vi "Display_Module.vi"(6 "Start pixel for display":i32=1, 7 "FOV: #A-lines":i32=2048, 8 "error in":errorcluster, 9 "Total pixels to display":i32=500, 10 "Source in":T1) -> (0 "error out":errorcluster, 2 "Image":T1(plugin-control))   [LabVIEW 2018]
uses:
  <vilib>/vision/Image Controls.llb/IMAQ Image.ctl
  Controls/Queue Manager Actions.ctl
  <vilib>/vision/NI_Vision_Development_Module.lvlib
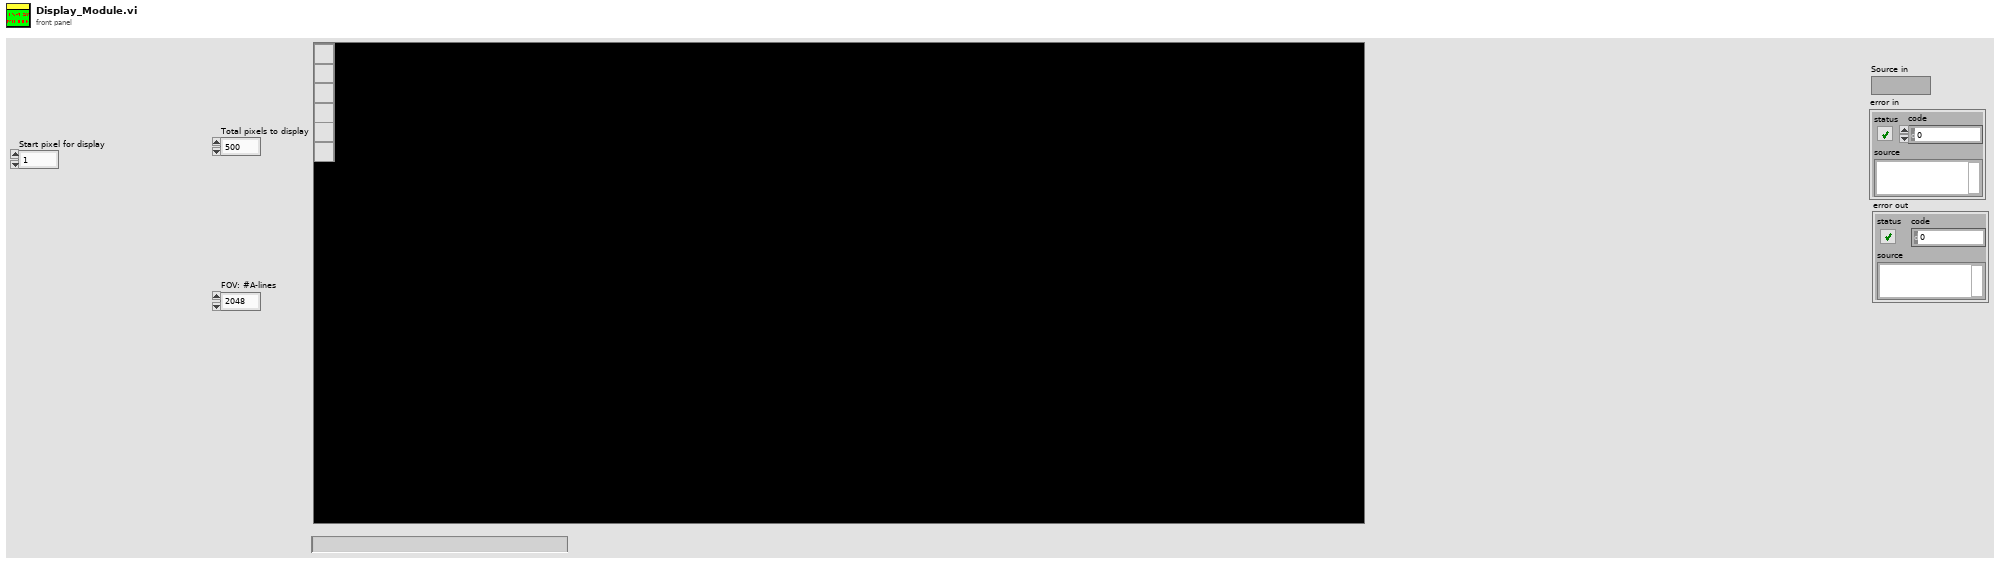
[diagram p1: front panel]
types:
  T1 = typedef "IMAQ Image.ctl" = refnum<image>
  T2 = typedef "Queue Manager Actions.ctl" = enum16{"Init", "Enqueue", "Enqueue All", "Preview Queue", "Dequeue", "Get Status", "Flush Queue", "Flush All Queues", "Release All Queues", "Release Queue", "Enqueue at Opposite End"}
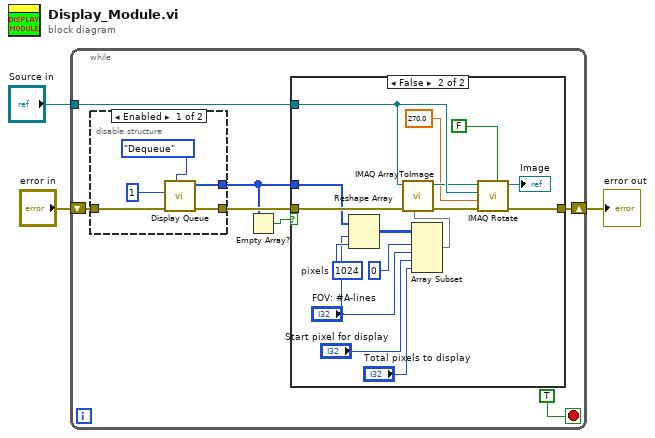
[diagram p0: block diagram]
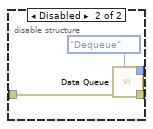
[diagram p3: hidden frame]
diagram:
  n1 = while {
    tunnel: "Source in" -> [w9]
    shift-right: [w8] -> w1
    shift-left: "error in" -> [w6]
    stop <- TRUE stop-if-true
    n2 = disable-structure shown="Enabled" {
      disable-tunnel: [w32 w35] -> w10
      disable-tunnel: [w29 w33] -> w4
      disable-tunnel: w6 -> [w28 w36]
      frame Enabled {
        n3 = call "Display Queue.vi"("Action"=Queue_Manager_Actions."Dequeue", "error in (no error)"=w28, "time out"=1) -> ("error out"=w32:errorcluster, "output data"=w29:u16[])  [unwired: 4 in, 3 out]
      }
      frame Disabled {
        n4 = call "Data Queue.vi"("Action"=Queue_Manager_Actions."Dequeue", "error in (no error)"=w36) -> ("error out"=w35:errorcluster, "data out"=w33:u16[])  [unwired: 7 in, 1 out]
      }
    }
    n5 = Empty Array?(array=w4) -> (empty?=w5:bool)
    n6 = case shown="False" w5 {
      tunnel: w10 -> [w11 w27]
      tunnel: w9 -> [_ w26]
      tunnel: [w11 w25] -> w8
      tunnel: w4 -> [_ w24]
      frame True {
      }
      frame False {
        w23 = 1024  # pixels
        n7 = Reshape Array(w24, "FOV: #A-lines", w23) -> (w13:u16[][])
        n8 = Array Subset(array=w13, index (row)=0 ("index"), length (row)="FOV: #A-lines", index (col)="Start pixel for display", length (col)="Total pixels to display") -> (w12:u16[][])
        n9 = call "IMAQ ArrayToImage"("Image Pixels (Float)"=w12, "error in (no error)"=w27, "Image"=w26) -> ("error out"=w21:errorcluster, "Image Out"=w22:T1)  [unwired: 7 in]
        n10 = call "IMAQ Rotate"("Maintain Size"=FALSE, "error in (no error)"=w21, "Angle (degrees)"=sgl 270.0, "Image Dst"=w26, "Image Src"=w22) -> ("error out"=w25:errorcluster, "Image Dst Out"=→"Image":T1)  [unwired: 5 in]
      }
    }
  }
  "error out" <- w1
